vi "DB-连接.vi"(7 "超时(5)":i32=5, 11 "DB路径":path) -> (0 "error out":errorcluster, 3 "connection reference":T1)   [LabVIEW 2017]
uses:
  <vilib>/addons/database/Connection.llb/Conn ObjectReference.ctl
  <vilib>/addons/database/Connection.llb/DB Tools Open Connec (String).vi
  <vilib>/addons/database/NI_Database_API.lvlib
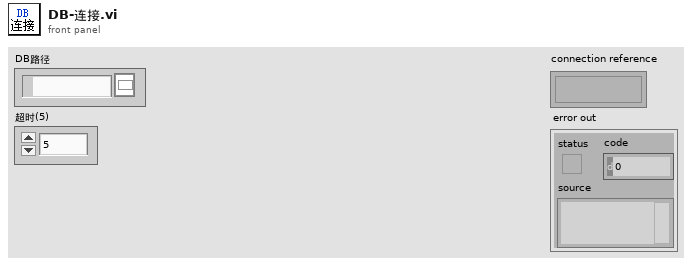
[diagram p1: front panel]
types:
  T1 = typedef "NI_Database_API.lvlib/Conn ObjectReference.ctl" = refnum<k1>
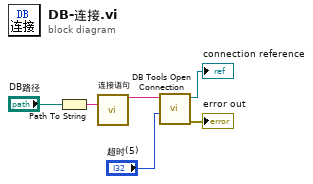
[diagram p0: block diagram]
diagram:
  n1 = Path To String(path="DB路径") -> (string=w3:string)
  n2 = call "连接语句"("文件路径"=w3) -> ("Result"=w6:string)  [unwired: 13 in, 1 out]
  n3 = call-poly <vilib>:"DB Tools Open Connection.vi"("connection timeout (15)"="超时(5)", "connection information"=w6) -> ("error out"=→"error out":errorcluster, "connection reference"=→"connection reference":T1)  [unwired: 6 in]
